vi "Set Root Element.vi"(8 "error in (no error)":errorcluster, 10 "Config Element":refnum<class "Config Element.lvclass">, 11 "Config Storage in":refnum<class "Config Storage.lvclass">) -> (0 "error out":errorcluster, 3 "Config Storage out":refnum<class "Config Storage.lvclass">)   [LabVIEW 2020, in "CDM-Config.lvlib" / "Config Storage.lvclass"]
uses:
  Config Storage.lvclass
  Config Element/Config Element.lvclass
  Config Storage.lvclass/Config Storage.ctl
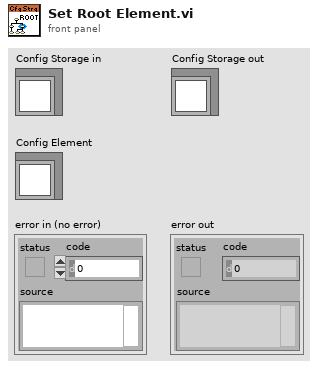
[diagram p1: front panel]
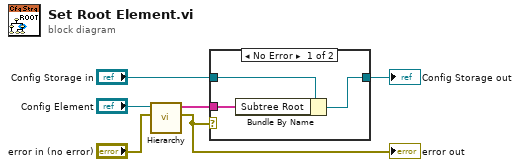
[diagram p0: block diagram]
diagram:
  n1 = call "Hierarchy.vi"("error in (no error)"="error in (no error)", "Config Element in"="Config Element") -> ("error out"=w1:errorcluster, "Hierarchy"=w5:string[])  [unwired: 8 in]
  "error out" <- w1
  n2 = case shown="No Error" w1 {
    tunnel: w5 -> [w9 _]
    tunnel: "Config Storage in" -> [w8 w10]
    tunnel: [w7 w10] -> w2
    frame No Error {
      n3 = Bundle By Name(cluster=w8, "Subtree Root"=w9) -> (w7:refnum<class "Config Storage.lvclass">)
    }
    frame Error {
    }
  }
  "Config Storage out" <- w2
